vi "ShearRampConfigUI .vi"() -> (1 "Confirmed?":bool, 3 "ShearRampConfiguration":T1={"Shear Ramp"="Linear", "Rotation or Torque"="Rotation (RPM)", "Initial Value"=0.0, "Final Value"=0.0, "Duration"=0.0, "Number of Points"=0, "Confirmed?"=FALSE, "Shear Ramp Array"=[]})   [LabVIEW 2021]
uses:
  TypeDefs/ShearRampConfiguration.ctl
  <vilib>/Analysis/1siggen.llb/Ramp Pattern by Samples.vi
  <vilib>/Analysis/NI_AALBase.lvlib
panel:
  out "Waveform Graph":waveform(dbl)(graph)
  in  "Visualize":bool
  in  "Number of Points":i32
  in  "Shear Ramp":string(combo)="Linear"
  in  "Final Value":dbl
  in  "Duration":dbl caption="Duration (s)"
  in  "Rotation or Torque":string(combo)="Rotation (RPM)"
  in  "Cancel":bool
  in  "Confirm button":bool
  in  "Initial Value":dbl
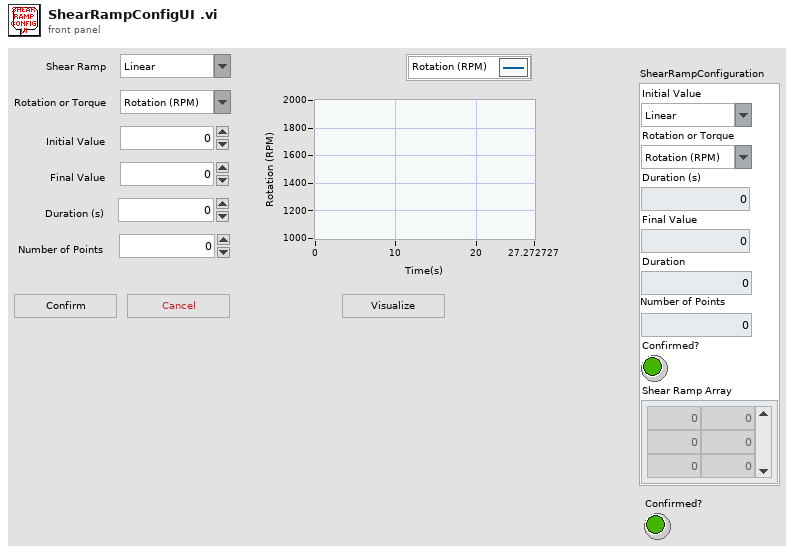
[diagram p1: front panel]
types:
  T1 = typedef "ShearRampConfiguration.ctl" = cluster{"Shear Ramp":string, "Rotation or Torque":string, "Initial Value":dbl, "Final Value":dbl, "Duration":dbl, "Number of Points":i32, "Confirmed?":bool, "Shear Ramp Array":dbl[][]}
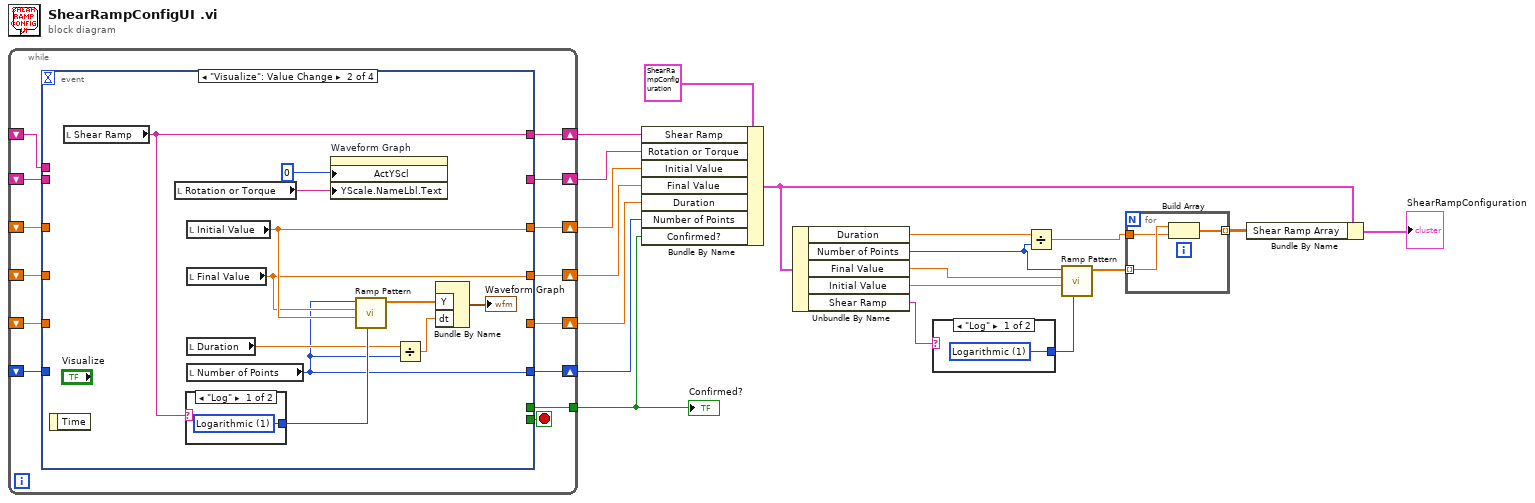
[diagram p0: block diagram]
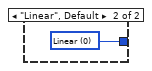
[diagram p2: hidden frame]
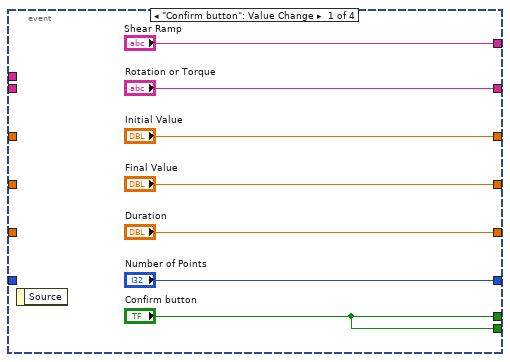
[diagram p3: hidden frame]
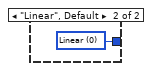
[diagram p4: hidden frame]
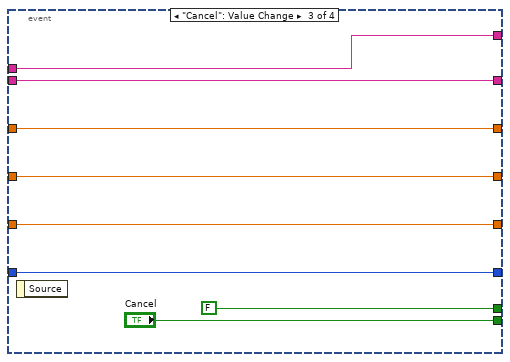
[diagram p5: hidden frame]
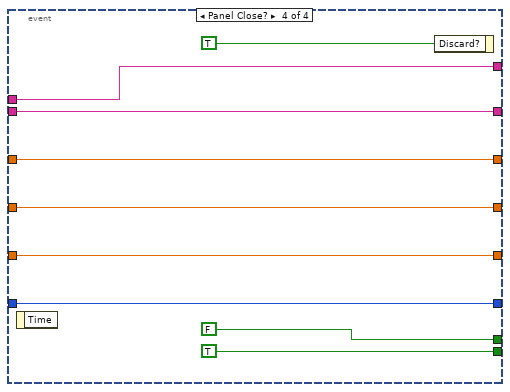
[diagram p6: hidden frame]
diagram:
  n1 = while {
    shift-right: [w33] -> w16
    shift-left: _ -> [w31]
    shift-right: [w32] -> w19
    shift-left: _ -> [w30]
    tunnel: [w29] -> w4
    shift-right: [w27] -> w17
    shift-left: _ -> [w26]
    shift-right: [w25] -> w15
    shift-left: _ -> [w24]
    shift-right: [w23] -> w14
    shift-left: _ -> [w22]
    shift-right: [w21] -> w13
    shift-left: _ -> [w20]
    stop <- w28 stop-if-true
    n2 = event shown="[1] \"Visualize\": Value Change" {
      selector: _ -> [_ _ _ _]
      dyn-events: _ -> [_ _ _ _]
      timeout: _ -> [_ _ _ _]
      tunnel: ["Initial Value" w49 w61 w67] -> w33
      tunnel: ["Rotation or Torque" _ w59 w66] -> w32
      tunnel: w31 -> [_ _ w61 w67]
      tunnel: w30 -> [_ _ w59 w66]
      tunnel: ["Confirm button" _ FALSE ("Confirm button") FALSE ("Confirm button")] -> w29
      tunnel: ["Confirm button" _ "Cancel" TRUE ("Cancel")] -> w28
      tunnel: ["Duration" _ w57 w65] -> w27
      tunnel: w26 -> [_ _ w57 w65]
      tunnel: ["Final Value" w48 w56 w64] -> w25
      tunnel: w24 -> [_ _ w56 w64]
      tunnel: ["Shear Ramp" w46 w55 w63] -> w23
      tunnel: w22 -> [_ _ w55 w63]
      tunnel: ["Number of Points" w41 w54 w62] -> w21
      tunnel: w20 -> [_ _ w54 w62]
      event "Confirm button": Value Change {
        n3 = event-data() -> ()  [unwired: 1 in, 1 out]
      }
      event "Visualize": Value Change {
        n4 = event-data() -> ()  [unwired: 1 in, 1 out]
        n5 = local read "Shear Ramp"() -> (w46:string)
        n6 = local read "Rotation or Torque"() -> (w45:string)
        n7 = case shown="\"Log\"" w46 {
          tunnel: [w52 w53] -> w47
          frame "Log" {
            w52 = u16 1 items=["Linear", "Logarithmic"] ("type")
          }
          frame "Linear", Default {
            w53 = u16 0 items=["Linear", "Logarithmic"] ("type")
          }
        }
        n8 = local read "Initial Value"() -> (w49:dbl)
        n9 = local read "Final Value"() -> (w48:dbl)
        n10 = local read "Duration"() -> (w43:dbl)
        n11 = local read "Number of Points"() -> (w41:i32)
        n12 = property on="Waveform Graph" class="WFGraph (strict)"("ActYScl"=0 ("Active Y Scale"), "YScale.NameLbl.Text"=w45) -> ()  [unwired: 2 in, 2 out]
        n13 = call-poly <vilib>:"Ramp Pattern.vi"("type"=w47, "start"=w49, "end"=w48, "samples"=w41) -> ("Ramp Pattern"=w50:dbl[])  [unwired: 6 in, 1 out]
        n14 = Divide(x=w43, y=w41) -> (x/y=w42:dbl)
        n15 = Bundle By Name("Y"=w50, "dt"=w42) -> (→"Waveform Graph":waveform(dbl))  [unwired: 1 in]
      }
      event "Cancel": Value Change {
        n16 = event-data() -> ()  [unwired: 1 in, 1 out]
      }
      event Panel Close? {
        n17 = event-data() -> ()  [unwired: 1 in, 1 out]
        n18 = event-data("Discard?"=TRUE) -> ()  [unwired: 1 in, 1 out]
      }
    }
  }
  "Confirmed?" <- w4
  n19 = Bundle By Name(cluster=T1 {"Shear Ramp"="Linear", "Rotation or Torque"="Rotation (RPM)", "Initial Value"=0.0, "Final Value"=0.0, "Duration"=0.0, "Number of Points"=0, "Confirmed?"=FALSE, "Shear Ramp Array"=[]} ("ShearRampConfiguration"), "Shear Ramp"=w14, "Rotation or Torque"=w19, "Initial Value"=w16, "Final Value"=w15, "Duration"=w17, "Number of Points"=w13, "Confirmed?"=w4) -> (w8:T1)
  n20 = Unbundle By Name(w8) -> ("Duration"=w3:dbl, "Number of Points"=w2:i32, "Final Value"=w12:dbl, "Initial Value"=w11:dbl, "Shear Ramp"=w10:string)
  n21 = case shown="\"Log\"" w10 {
    tunnel: [w71 w72] -> w9
    frame "Log" {
      w71 = u16 1 items=["Linear", "Logarithmic"] ("type")
    }
    frame "Linear", Default {
      w72 = u16 0 items=["Linear", "Logarithmic"] ("type")
    }
  }
  n22 = Divide(x=w3, y=w2) -> (x/y=w1:dbl)
  n23 = call-poly <vilib>:"Ramp Pattern.vi"("type"=w9, "start"=w11, "end"=w12, "samples"=w2) -> ("Ramp Pattern"=w5:dbl[])  [unwired: 6 in, 1 out]
  n24 = for {
    tunnel: w5 -> [w75] mode=indexing
    tunnel: w1 -> [w73]
    tunnel: [w74] -> w6 mode=indexing
    n25 = Build Array(w75, w73) -> (w74:dbl[])
  }
  n26 = Bundle By Name(cluster=w8, "Shear Ramp Array"=w6) -> (→"ShearRampConfiguration":T1)
